vi "Measure_Voltage.vi"(8 "error in (no error)":errorcluster, 10 "Measure_Configuration":variant, 11 "Measure_Voltage in":refnum<class "Measure_Voltage.lvclass">) -> (0 "error out":errorcluster, 1 "Out of Range":bool, 2 "DC_Voltage":dbl, 3 "Measure_Voltage out":refnum<class "Measure_Voltage.lvclass">)   [LabVIEW 2020, in "Measure_Voltage.lvclass"]
uses:
  Measure_Voltage.lvclass
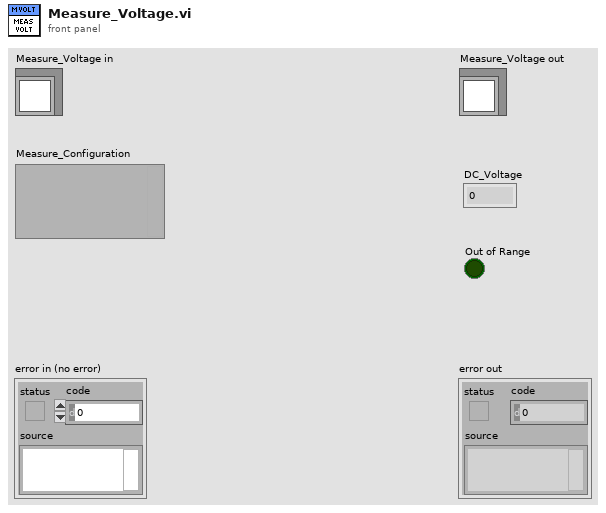
[diagram p1: front panel]
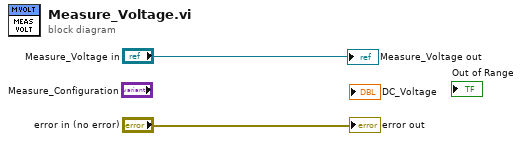
[diagram p0: block diagram]
diagram:
  "error out" <- "error in (no error)"
  "Measure_Voltage out" <- "Measure_Voltage in"
